vi "Copy File(s) with Ask - CORE.vi"(6 "Use Prev Answer":bool, 7 "Prev Answer":T1=enum."Copy", 8 "Error In":errorcluster, 9 "On File Coillision":T2={"Dest is Newer & RO"=enum."Skip", "Dest is Newer & RW"=enum."Skip", "Dest is Older & RO"=enum."Ask", "Dest is Older & RW"=enum."Overwrite Siliently"}, 10 "Destination Foilder":path, 11 "Source File":path) -> (0 "Error Out":errorcluster, 3 "New Path":path, 4 "Use same answer for all":bool, 5 "Answer":T1=enum."Copy")   [LabVIEW 2018]
doc: "Copies a set of files to a folder. Retains file hierarchy based on common node of input file paths.\nOptions for file collisions:\n Throw Error\n Ask\n Ask if Source is Older\n Skip\n Skip if Source is Older\n Overwrite Silently"
uses:
  File Collision Options.ctl
  Dialog Buttons.ctl
  <vilib>/Utility/error.llb/Error Cluster From Error Code.vi
  <vilib>/ErrorRing/Error Ring.xnode
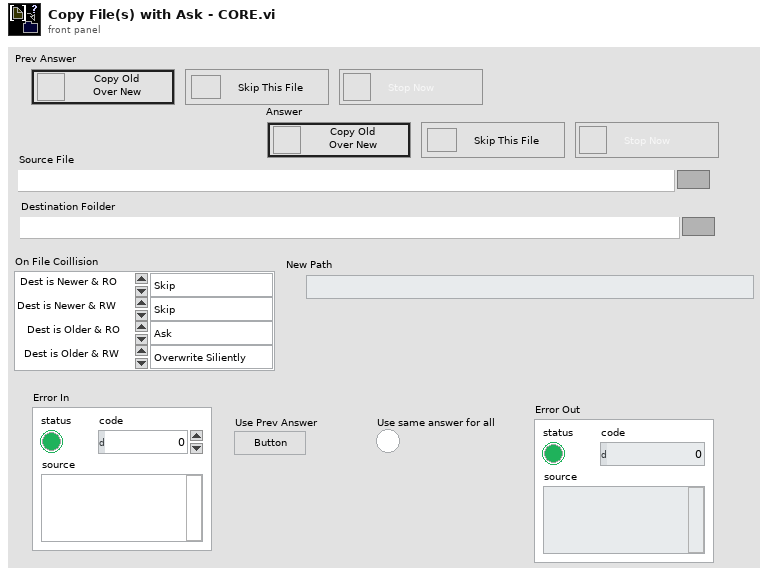
[diagram p1: front panel]
types:
  T1 = typedef "Dialog Buttons.ctl" = enum32{"No Selection", "Copy", "Skip Ahead", "Stop"}
  T2 = typedef "File Collision Options.ctl" = cluster{"Dest is Newer & RO":enum16{"Throw Error", "Ask", "Skip", "Overwrite Siliently"}, "Dest is Newer & RW":enum16{"Throw Error", "Ask", "Skip", "Overwrite Siliently"}, "Dest is Older & RO":enum16{"Throw Error", "Ask", "Skip", "Overwrite Siliently"}, "Dest is Older & RW":enum16{"Throw Error", "Ask", "Skip", "Overwrite Siliently"}}
  T3 = enum16{"Throw Error", "Ask", "Skip", "Overwrite Siliently"}
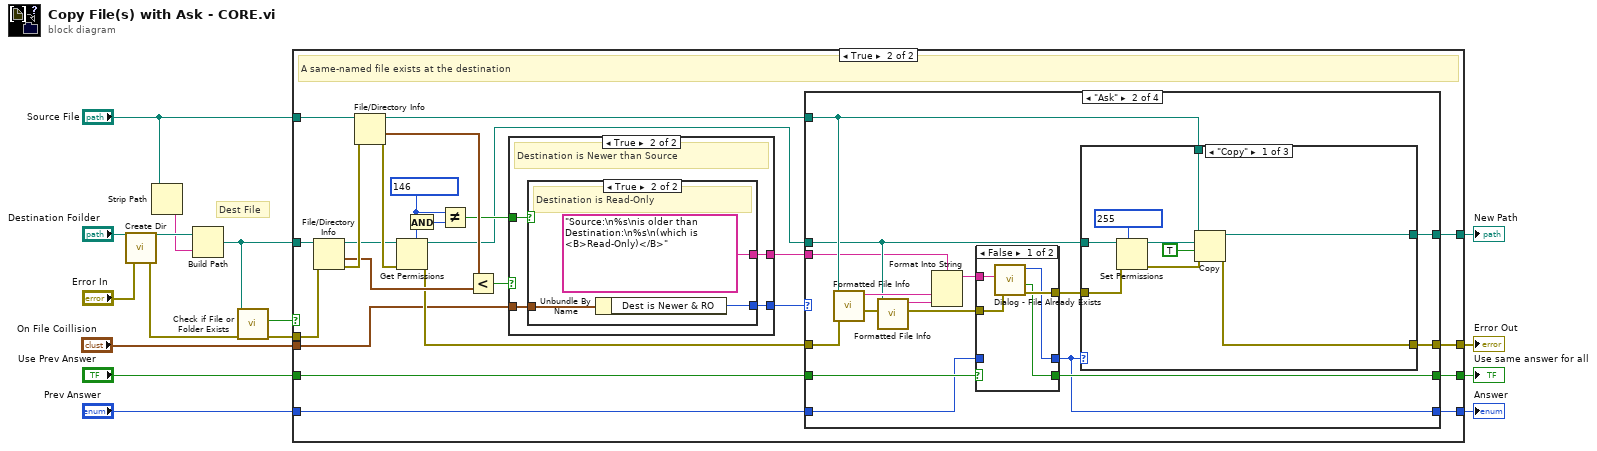
[diagram p0: block diagram]
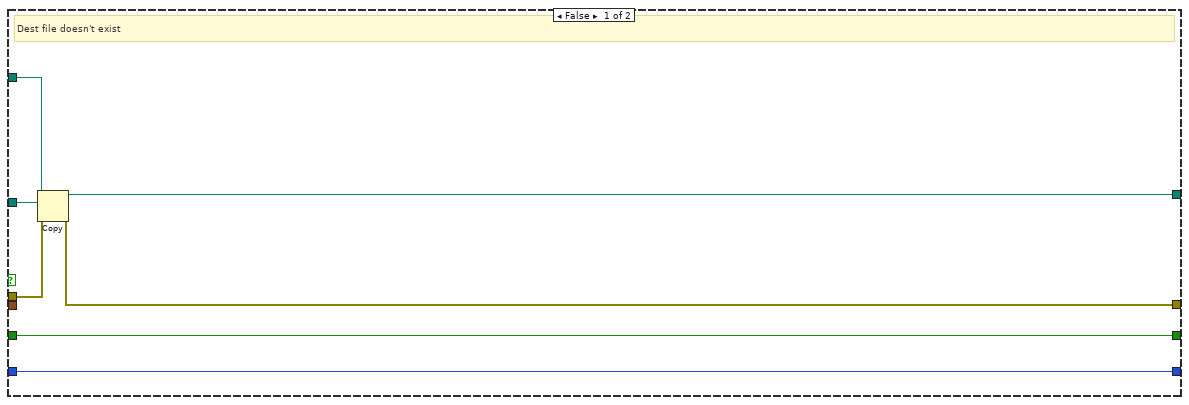
[diagram p2: hidden frame]
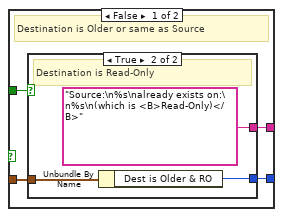
[diagram p3: hidden frame]
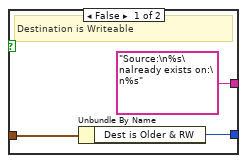
[diagram p4: hidden frame]
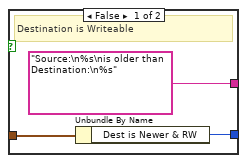
[diagram p5: hidden frame]
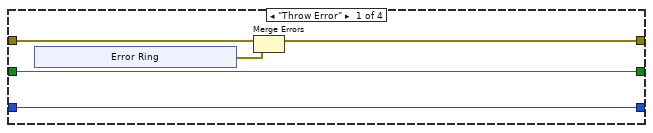
[diagram p6: hidden frame]
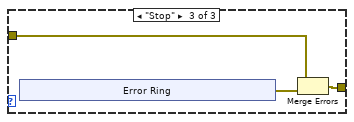
[diagram p9: hidden frame]
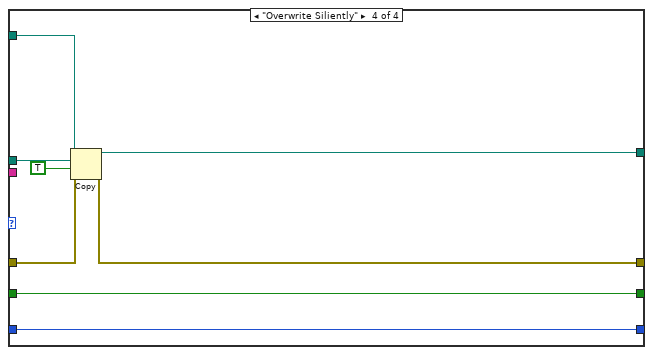
[diagram p11: hidden frame]
diagram:
  # "Dest File"
  n1 = call "Create Dir.vi"("error in"="Error In", "path"="Destination Foilder") -> ("error out"=w4:errorcluster, "path out"=w8:path)  [unwired: 4 in]
  n2 = Strip Path(path="Source File") -> (name=w6:string)  [unwired: 1 out]
  n3 = Build Path(base path=w8, name or relative path=w6) -> (appended path=w11:path)
  n4 = call <vilib>:"Check if File or Folder Exists.vi"("error in (no error)"=w4, "path"=w11) -> ("error out"=w12:errorcluster, "file or folder exists?"=w13:bool)  [unwired: 7 in, 1 out]
  n5 = case shown="True" w13 {
    tunnel: w11 -> [w20 w38]
    tunnel: "Source File" -> [w19 w40]
    tunnel: w12 -> [w23 w43]
    tunnel: "On File Coillision" -> [_ w28]
    tunnel: [w22 w48] -> w14
    tunnel: [w21 w47] -> w10
    tunnel: "Use Prev Answer" -> [w21 w46]
    tunnel: "Prev Answer" -> [w18 w32]
    tunnel: [w18 w31] -> w2
    tunnel: [w17 w24] -> w1
    frame False {
      # "Dest file doesn't exist"
      n6 = Copy(8:w23, 10:w20, 11:w19) -> (0:w22:errorcluster, 3:w17:path)  [unwired: 2 in, 1 out]
    }
    frame True {
      w33 = i16 146 ("x")
      # "A same-named file exists at the destination"
      n7 = File/Directory Info(path=w38, error in=w43) -> (path out=w39:path, last mod=w37:timestamp, error out=w45:errorcluster)  [unwired: 4 out]
      n8 = File/Directory Info(path=w40, error in=w45) -> (path out=w41:path, last mod=w44:timestamp, error out=w42:errorcluster)  [unwired: 4 out]
      n9 = Get Permissions(8:w42, 11:w39) -> (0:w36:errorcluster, 3:w27:path, 5:w35:i16)  [unwired: 2 out]
      n10 = And(x=w33, y=w35) -> (x .and. y?=w34:i16)
      n11 = Not Equal?(x=w33, y=w34) -> (x != y?=w30:bool)
      n12 = Less?(x=w44, y=w37) -> (x < y?=w29:bool)
      n13 = case shown="True" w29 {
        tunnel: w30 -> [w52 w62]
        tunnel: w28 -> [w51 w61]
        tunnel: [w50 w60] -> w26
        tunnel: [w49 w59] -> w25
        frame False {
          # "Destination is Older or same as Source"
          n14 = case shown="True" w52 {
            tunnel: w51 -> [w55 w58]
            tunnel: [w54 w57] -> w50
            tunnel: ["Source:\n%s\nalready exists on:\n%s" ("format string") "Source:\n%s\nalready exists on:\n%s\n(which is <B>Read-Only)</B>" ("format string")] -> w49
            frame False {
              # "Destination is Writeable"
              n15 = Unbundle By Name(w55) -> ("Dest is Older & RW"=w54:T3)
            }
            frame True {
              # "Destination is Read-Only"
              n16 = Unbundle By Name(w58) -> ("Dest is Older & RO"=w57:T3)
            }
          }
        }
        frame True {
          # "Destination is Newer than Source"
          n17 = case shown="True" w62 {
            tunnel: w61 -> [w65 w68]
            tunnel: [w64 w67] -> w60
            tunnel: ["Source:\n%s\nis older than Destination:\n%s" ("format string") "Source:\n%s\nis older than Destination:\n%s\n(which is <B>Read-Only)</B>" ("format string")] -> w59
            frame False {
              # "Destination is Writeable"
              n18 = Unbundle By Name(w65) -> ("Dest is Newer & RW"=w64:T3)
            }
            frame True {
              # "Destination is Read-Only"
              n19 = Unbundle By Name(w68) -> ("Dest is Newer & RO"=w67:T3)
            }
          }
        }
      }
      n20 = case shown="\"Ask\"" w26 {
        tunnel: w41 -> [_ w86 _ w125]
        tunnel: w27 -> [_ w85 _ w126]
        tunnel: [w72 w93 w120 w129] -> w48
        tunnel: [w71 w83 w121 w128] -> w47
        tunnel: w46 -> [w71 w82 w121 w128]
        tunnel: w36 -> [w70 w84 w120 w124]
        tunnel: w32 -> [w69 w81 w119 w123]
        tunnel: [w69 w80 w119 w123] -> w31
        tunnel: w25 -> [_ w78 _ _]
        tunnel: [_ w79 _ w122] -> w24
        frame "Throw Error" {
          n21 = xnode "Error Ring"() -> ("error out"=w73:errorcluster)
          n22 = Merge Errors(w70, w73) -> (w72:errorcluster)
        }
        frame "Ask" {
          n23 = call "Formatted File Info.vi"("Path"=w86, "Error In"=w84) -> ("Formatted String"=w90:string, "Error Out"=w88:errorcluster)  [unwired: 4 in]
          n24 = call "Formatted File Info.vi"("Path"=w85, "Error In"=w88) -> ("Formatted String"=w89:string, "Error Out"=w87:errorcluster)  [unwired: 4 in]
          n25 = Format Into String(format string=w78, w90, w89) -> (resulting string=w92:string)  [unwired: 2 in, 1 out]
          n26 = case shown="False" w82 {
            selector: w82 -> [_ w100]
            tunnel: w92 -> [w98 _]
            tunnel: [w97 w101] -> w91
            tunnel: w87 -> [w96 w101]
            tunnel: [w95 w100] -> w83
            tunnel: [w94 w99] -> w80
            tunnel: w81 -> [_ w99]
            frame False {
              n27 = call "Dialog - File Already Exists.vi"("Error In"=w96, "Message In"=w98) -> ("Error Out"=w97:errorcluster, "Do same for all"=w95:bool, "Selected Button"=w94:T1)  [unwired: 3 in]
            }
            frame True {
            }
          }
          n28 = case shown="\"Copy\"" w80 {
            tunnel: w86 -> [w107 _ _]
            tunnel: w85 -> [w108 _ _]
            tunnel: w91 -> [w103 w111 w112]
            tunnel: [w110 w111 w113] -> w93
            tunnel: [w106 _ _] -> w79
            frame "Copy" {
              n29 = Set Permissions(7:i16 255 ("permissions"), 8:w103, 11:w108) -> (0:w104:errorcluster, 3:w105:path)  [unwired: 2 in]
              n30 = Copy(8:w104, 9:TRUE ("overwrite (F)"), 10:w105, 11:w107) -> (0:w110:errorcluster, 3:w106:path)  [unwired: 1 in, 1 out]
            }
            frame "No Selection", "Skip Ahead" {
            }
            frame "Stop" {
              n31 = xnode "Error Ring"() -> ("error out"=w114:errorcluster)
              n32 = Merge Errors(w112, w114) -> (w113:errorcluster)
            }
          }
        }
        frame "Skip" {
        }
        frame "Overwrite Siliently" {
          n33 = Copy(8:w124, 9:TRUE ("overwrite (F)"), 10:w126, 11:w125) -> (0:w129:errorcluster, 3:w122:path)  [unwired: 1 in, 1 out]
        }
      }
    }
  }
  "Error Out" <- w14
  "Answer" <- w2
  "Use same answer for all" <- w10
  "New Path" <- w1
